vi "SetAutoReconnectTimes.vi"(0 "reference in":refnum<class "VdTcpIP.lvclass">, 1 "AutoReConnectTimes":i32, 3 "AutoReConnectInterval(100ms)":i32=100, 5 "error in (no error)":errorcluster) -> (14 "reference out":refnum<class "VdTcpIP.lvclass">, 19 "error out":errorcluster)   [LabVIEW 2020, in "VdTcpIP.lvclass"]
uses:
  VdTcpIP.lvclass
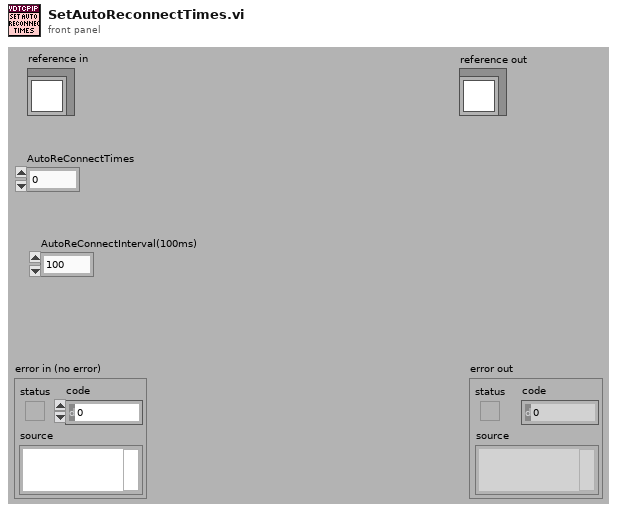
[diagram p1: front panel]
types:
  T1 = typedef "VdTcpIP.lvclass/ObjectAttributes.ctl" = cluster{"IP-Address":string, "Port":u16, "Connection":refnum<k5>, "Listener":refnum<k5>, "ListenerConnection":refnum<k5>, "Listner":bool, "ListnerProcessRunning":bool, "InConnections":refnum<k5>[], "InConnectionsIP":string[], "InConnectionAdded":refnum<notifier>, "RunVIOnNewConnection":variant, "DataToNewConnectionVI":cluster{"ControlName":string, "ControlValue":variant}[], "WebServicesURL_Location(http://...)":string, "WebServicesPostWebPage(*.asmx)":string, "Semaphore":T2, "AutoReConnectTimes":i32, "AutoReConnectInterval(ms)":i32, "ConnectionTimeout":i32}
  T2 = typedef "Semaphore RefNum" = refnum<k1>
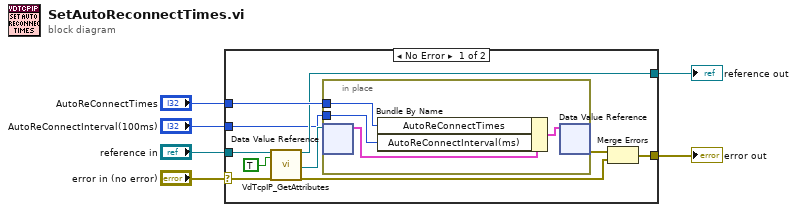
[diagram p0: block diagram]
diagram:
  n1 = case shown="No Error" "error in (no error)" {
    selector: "error in (no error)" -> [w10 w22]
    tunnel: [w14 w22] -> w5
    tunnel: [w12 w21] -> w3
    tunnel: "reference in" -> [w13 w21]
    tunnel: "AutoReConnectTimes" -> [w16 _]
    tunnel: "AutoReConnectInterval(100ms)" -> [w7 _]
    frame No Error {
      n2 = call "VdTcpIP_GetAttributes.vi"("reference in"=w13, "OnlyGetDvrReference(False)"=TRUE, "error in (no error)"=w10) -> ("reference out"=w12:refnum<class "VdTcpIP.lvclass">, "DataRef"=w11:refnum<data-value>, "error out"=w9:errorcluster)  [unwired: 13 in, 1 out]
      n3 = in-place {
        in-place-border: w16 -> [w20]
        in-place-border: w7 -> [w17]
        n4 = in-place-dvr #1(w11) -> (w19:T1)  [unwired: 1 out]
        n5 = Bundle By Name(cluster=w19, "AutoReConnectTimes"=w20, "AutoReConnectInterval(ms)"=w17) -> (w18:T1)
        n6 = in-place-dvr #1(w18) -> (w15:errorcluster)  [unwired: 1 out]
      }
      n7 = Merge Errors(w15, w9) -> (w14:errorcluster)
    }
    frame Error {
    }
  }
  "error out" <- w5
  "reference out" <- w3
